vi "Convert to AutonEnum.vi"(11 "Auton In":T1) -> (3 "Auton Out":T1)   [LabVIEW 2014]
uses:
  Lightning base/Auton Modes.ctl
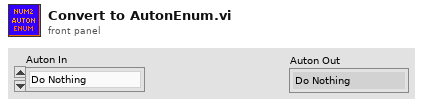
[diagram p1: front panel]
types:
  T1 = typedef "Auton Modes.ctl" = enum16{"Do Nothing", "Snake", "Move Forward", "Move Forward w/Tote", "Move Forward w/RC", "Gather RC from Step", "3 Tote Auton", "Vision Test", "Strafer"}
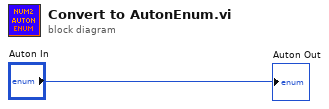
[diagram p0: block diagram]
diagram:
  "Auton Out" <- "Auton In"
